vi "Dialogue_Password.vi"(8 "error in":errorcluster, 11 "Title":string) -> (0 "error out":errorcluster, 1 "Cancelled?":bool, 2 "Password OUT":string)   [LabVIEW 2022 SP3, in "hse-ui.lvlib"]
doc: "Shows a dialog window for entering a password.\n\n____\nHAMPEL SOFTWARE ENGINEERING v3.8.0 (2023-12-18 14:41)"
uses:
  hse-ui.lvlib
  FPControl/FPControl_Actions.ctl
panel:
  in  "Password":string
  in  "Btn_Cancel":bool
  in  "Btn_OK":bool
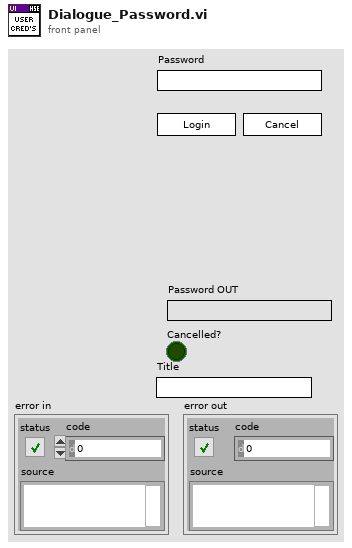
[diagram p1: front panel]
types:
  T1 = typedef "hse-ui.lvlib/FPControl_Actions.ctl" = enum16{"Open", "Hide", "Close", "Bring To Front", "Center", "Minimize", "Maximize"}
  T2 = enum8{"Enabled", "Disabled", "Disabled and Grayed Out"}
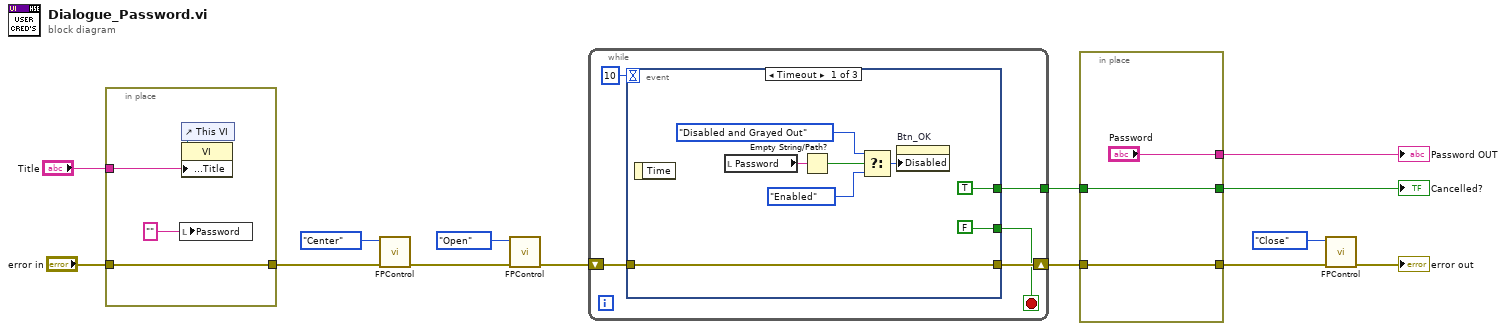
[diagram p0: block diagram]
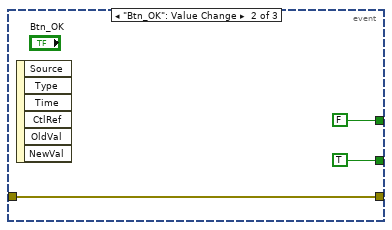
[diagram p2: hidden frame]
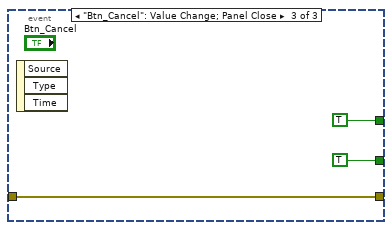
[diagram p3: hidden frame]
diagram:
  n1 = in-place {
    in-place-border: "error in" -> [w17]
    in-place-border: [w17] -> w8
    in-place-border: "Title" -> [w15]
    n2 = local write "Password"("" ("Username")) -> ()
    n3 = control-ref of="This VI"() -> (w16:refnum<vi>)
    n4 = property class="VI"(reference=w16, "Front Panel.Title"=w15) -> ()  [unwired: 1 in, 2 out]
  }
  n5 = call "FPControl.vi"("error in"=w8, "Function"=FPControl_Actions."Center") -> ("error out"=w12:errorcluster)  [unwired: 9 out]
  n6 = call "FPControl.vi"("error in"=w12, "Function"=FPControl_Actions."Open") -> ("error out"=w1:errorcluster)  [unwired: 9 out]
  n7 = while {
    shift-right: [w21] -> w7
    shift-left: w1 -> [w22]
    tunnel: [w19] -> w4
    stop <- w20 stop-if-true
    n8 = event shown="[0] Timeout" {
      selector: _ -> [_ _ _]
      dyn-events: _ -> [_ _ _]
      timeout: 10 -> [_ _ _]
      tunnel: w22 -> [w30 w34 w37]
      tunnel: [w30 w34 w37] -> w21
      tunnel: [FALSE TRUE TRUE] -> w20
      tunnel: [TRUE FALSE TRUE] -> w19
      event Timeout {
        n9 = event-data() -> ()  [unwired: 1 in, 1 out]
        n10 = local read "Password"() -> (w28:string)
        n11 = Empty String/Path?(string/path=w28) -> (empty?=w26:bool)
        n12 = Select(t=T2."Disabled and Grayed Out" ("Disabled"), s=w26, f=T2."Enabled" ("Disabled")) -> (s? t:f=w29:T2)
        n13 = property on="Btn_OK" class="Bool"("Disabled"=w29) -> ()  [unwired: 2 in, 2 out]
      }
      event "Btn_OK": Value Change {
        n14 = event-data() -> ()  [unwired: 1 in, 6 out]
      }
      event "Btn_Cancel": Value Change; Panel Close {
        n15 = event-data() -> ()  [unwired: 1 in, 3 out]
      }
    }
  }
  n16 = in-place {
    in-place-border: w7 -> [w40]
    in-place-border: [w40] -> w6
    in-place-border: [w39] -> w5
    in-place-border: w4 -> [w39]
    in-place-border: ["Password"] -> w3
  }
  "Cancelled?" <- w5
  "Password OUT" <- w3
  n17 = call "FPControl.vi"("error in"=w6, "Function"=FPControl_Actions."Close") -> ("error out"=→"error out":errorcluster)  [unwired: 9 out]
